vi "cityGridCoordinates.vi"(10 "Row":i32=3, 11 "Column":i32) -> (3 "Cluster":cluster{"x":dbl, "y":dbl})   [LabVIEW 2016]
panel:
  in  "Array":cluster{"x":dbl, "y":dbl}[][](array[cluster])=[[{"x"=1390.0, "y"=3700.0}, {"x"=2490.0, "y"=3700.0}, {"x"=3590.0, "y"=3700.0}, {"x"=4690.0, "y"=3700.0}], [{"x"=1390.0, "y"=2600.0}, {"x"=2490.0, "y"=2600.0}, {"x"=3590.0, "y"=2600.0}, {"x"=4690.0, "y"=2600.0}], [{"x"=1390.0, "y"=1500.0}, {"x"=2490.0, "y"=1500.0}, {"x"=3590.0, "y"=1500.0}, {"x"=4690.0, "y"=1500.0}]]
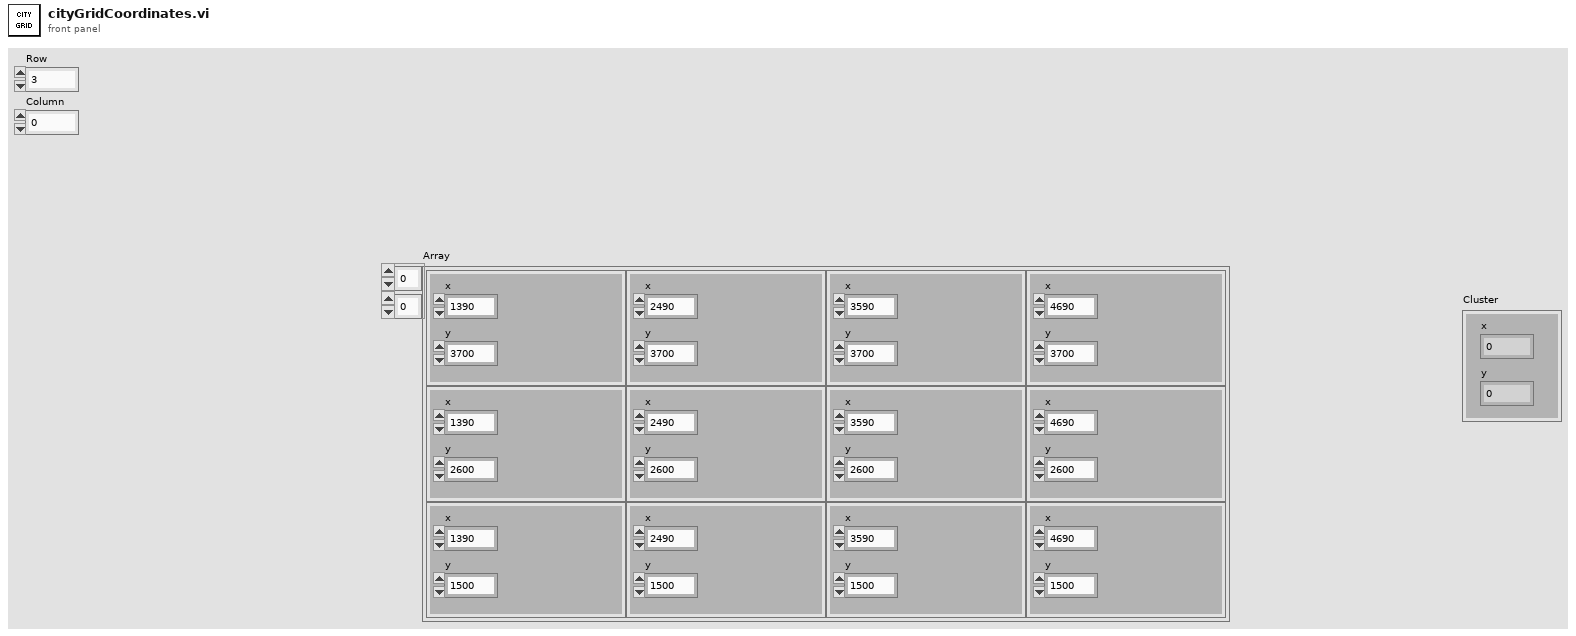
[diagram p1: front panel]
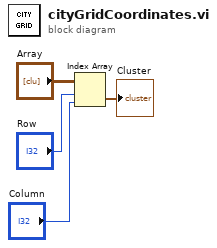
[diagram p0: block diagram]
diagram:
  n1 = Index Array(array="Array", index (row)="Row", index (col)="Column") -> (element=→"Cluster":cluster{"x":dbl, "y":dbl})
